vi "RSNRPZ Get Duty Cycle.vi"(8 "error in (no error)":errorcluster, 10 "Channel (1)":i32=1, 11 "VISA session":refnum<visa-resource-name> caption="VISA resource name") -> (0 "error out":errorcluster, 2 "Duty Cycle":dbl format="%.2p", 3 "dup VISA session":refnum<visa-resource-name> caption="VISA resource name")   [LabVIEW 2010]
doc: "This VI gets the size of duty cycle of the power to be measured.\n\nRemote-control command(s):\nSENS:CORR:DCYC?"
uses:
  rsnrpz_32.dll
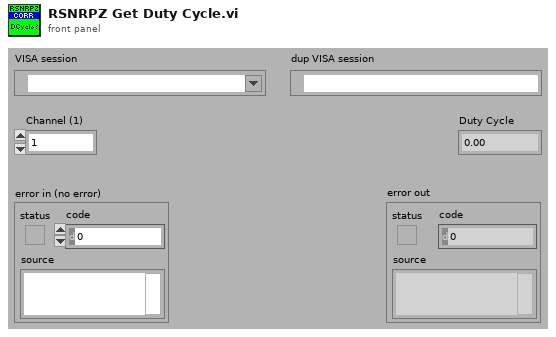
[diagram p1: front panel]
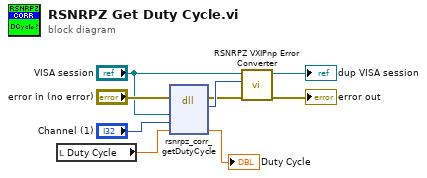
[diagram p0: block diagram]
diagram:
  n1 = local read "Duty Cycle"() -> (w7:dbl)
  n2 = dll-call lib="rsnrpz_32.dll" fn="rsnrpz_corr_getDutyCycle"(error in="error in (no error)", "VISA Session"="VISA session", "Channel"="Channel (1)", "Duty Cycle"=w7) -> (error out=w5:errorcluster, "Status"=w9:i32, "Duty Cycle"=→"Duty Cycle":dbl)  [unwired: 4 in, 1 out]
  n3 = call <instrlib>:"RSNRPZ VXIPnp Error Converter.vi"("error in"=w5, "VXIPnp error code"=w9, "VISA session"="VISA session") -> ("error out"=→"error out":errorcluster, "dup VISA session"=→"dup VISA session":refnum<visa-resource-name>)  [unwired: 7 in]
